vi "ASG example_By_CY.vi"() -> ()   [LabVIEW 2020]
uses:
  Labview Library/Libraries/ASG8100CY/ASG8X00_x64.dll
panel:
  out "连接状态":bool
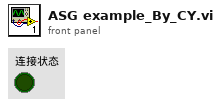
[diagram p1: front panel]
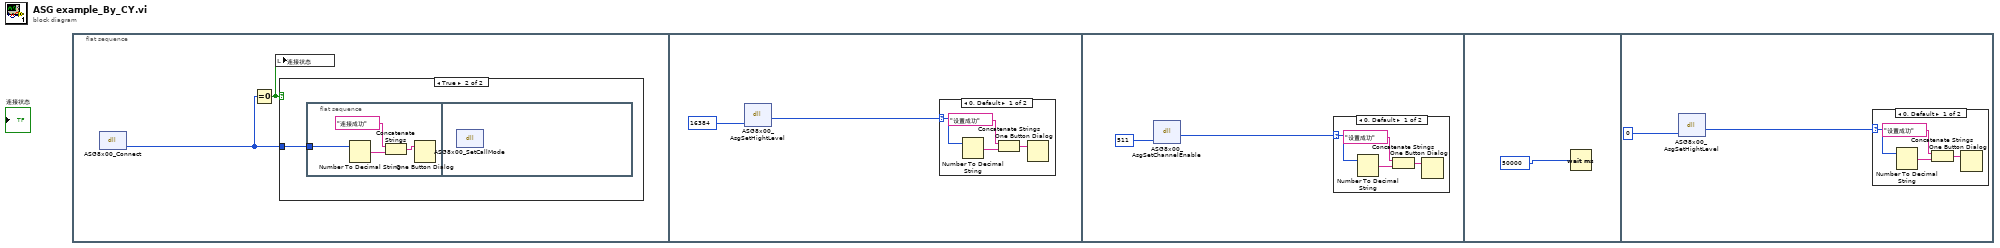
[diagram p0: block diagram]
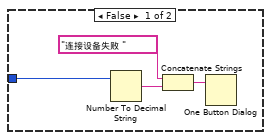
[diagram p2: hidden frame]
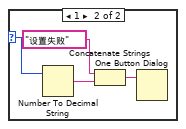
[diagram p3: hidden frame]
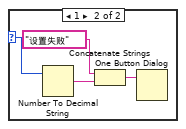
[diagram p4: hidden frame]
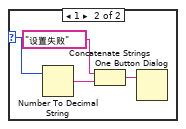
[diagram p5: hidden frame]
diagram:
  n1 = flat-sequence {
    frame #0 {
      n2 = dll-call lib="F:/Labview Library/Libraries/ASG8100CY/ASG8X00_x64.dll" fn="ASG8x00_Connect"() -> ("返回类型"=w2:i32)  [unwired: 3 in, 2 out]
      n3 = Equal To 0?(x=w2) -> (x = 0?=w1:bool)
      n4 = local write "连接状态"(w1) -> ()
      n5 = case shown="True" w1 {
        tunnel: w2 -> [w3 w7]
        frame False {
          n6 = Number To Decimal String(number=w3) -> (decimal integer string=w4:string)  [unwired: 1 in]
          n7 = Concatenate Strings("连接设备失败 ", w4) -> (w5:string)
          n8 = One Button Dialog(message=w5) -> ()  [unwired: 1 in, 1 out]
        }
        frame True {
          n9 = flat-sequence {
            tunnel: w7 -> [w8]
            frame #0 {
              n10 = Number To Decimal String ("数值至十进制数字符串转换")(number=w8) -> (decimal integer string=w10:string)  [unwired: 1 in]
              n11 = Concatenate Strings("连接成功", w10) -> (w11:string)
              n12 = One Button Dialog(message=w11) -> ()  [unwired: 1 in, 1 out]
            }
            frame #1 {
              n13 = dll-call lib="F:/Labview Library/Libraries/ASG8100CY/ASG8X00_x64.dll" fn="ASG8x00_SetCallMode"() -> ()  [unwired: 4 in, 2 out]
            }
          }
        }
      }
    }
    frame #1 {
      n14 = dll-call lib="F:/Labview Library/Libraries/ASG8100CY/ASG8X00_x64.dll" fn="ASG8x00_AsgSetHightLevel"("参数1"=16384) -> ("返回类型"=w13:i32)  [unwired: 4 in, 2 out]
      n15 = case shown="0, Default" w13 {
        selector: w13 -> [w14 w18]
        frame 0, Default {
          n16 = Number To Decimal String ("数值至十进制数字符串转换")(number=w14) -> (decimal integer string=w16:string)  [unwired: 1 in]
          n17 = Concatenate Strings("设置成功", w16) -> (w15:string)
          n18 = One Button Dialog(message=w15) -> ()  [unwired: 1 in, 1 out]
        }
        frame 1 {
          n19 = Number To Decimal String ("数值至十进制数字符串转换")(number=w18) -> (decimal integer string=w20:string)  [unwired: 1 in]
          n20 = Concatenate Strings("设置失败", w20) -> (w19:string)
          n21 = One Button Dialog(message=w19) -> ()  [unwired: 1 in, 1 out]
        }
      }
    }
    frame #2 {
      n22 = dll-call lib="F:/Labview Library/Libraries/ASG8100CY/ASG8X00_x64.dll" fn="ASG8x00_AsgSetChannelEnable"("参数1"=511) -> ("返回类型"=w23:i32)  [unwired: 4 in, 2 out]
      n23 = case shown="0, Default" w23 {
        selector: w23 -> [w24 w28]
        frame 0, Default {
          n24 = Number To Decimal String ("数值至十进制数字符串转换")(number=w24) -> (decimal integer string=w26:string)  [unwired: 1 in]
          n25 = Concatenate Strings("设置成功", w26) -> (w25:string)
          n26 = One Button Dialog(message=w25) -> ()  [unwired: 1 in, 1 out]
        }
        frame 1 {
          n27 = Number To Decimal String ("数值至十进制数字符串转换")(number=w28) -> (decimal integer string=w30:string)  [unwired: 1 in]
          n28 = Concatenate Strings("设置失败", w30) -> (w29:string)
          n29 = One Button Dialog(message=w29) -> ()  [unwired: 1 in, 1 out]
        }
      }
    }
    frame #3 {
      n30 = Wait (ms)(milliseconds to wait=50000) -> ()  [unwired: 1 out]
    }
    frame #4 {
      n31 = dll-call lib="F:/Labview Library/Libraries/ASG8100CY/ASG8X00_x64.dll" fn="ASG8x00_AsgSetHightLevel"("参数1"=0) -> ("返回类型"=w34:i32)  [unwired: 4 in, 2 out]
      n32 = case shown="0, Default" w34 {
        selector: w34 -> [w35 w39]
        frame 0, Default {
          n33 = Number To Decimal String ("数值至十进制数字符串转换")(number=w35) -> (decimal integer string=w37:string)  [unwired: 1 in]
          n34 = Concatenate Strings("设置成功", w37) -> (w36:string)
          n35 = One Button Dialog(message=w36) -> ()  [unwired: 1 in, 1 out]
        }
        frame 1 {
          n36 = Number To Decimal String ("数值至十进制数字符串转换")(number=w39) -> (decimal integer string=w41:string)  [unwired: 1 in]
          n37 = Concatenate Strings("设置失败", w41) -> (w40:string)
          n38 = One Button Dialog(message=w40) -> ()  [unwired: 1 in, 1 out]
        }
      }
    }
  }
